vi "FTW-Context-Instance.vi"() -> ()   [LabVIEW 2014, in "FTW-Actor-Context.lvclass"]
uses:
  FTW-Actor-Context.lvclass
  logger/FTW-Logger.lvclass
panel:
  in  "Application Version":string
  in  "Application Name":string
  in  "Logger Address":string
  in  "Default Linger":i32=500 format="%dmsec"
  in  "Logger":refnum<class "FTW-Logger.lvclass">
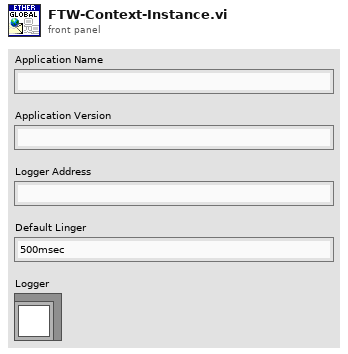
[diagram p1: front panel]
diagram:
